vi "BER_Graphic.vi"(4 "Window Size":dbl=30.0, 5 "Instantaneous BER":dbl) -> (2 "Graph Instantaneous BER":dbl)   [LabVIEW 2022 SP3]
uses:
  <vilib>/Analysis/baseanly.llb/Mean (DBL).vi
  <vilib>/Analysis/NI_AALBase.lvlib
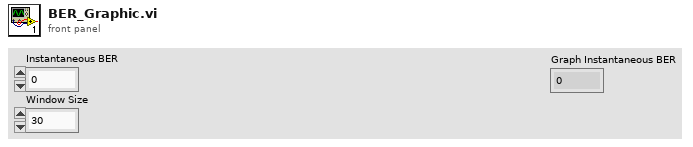
[diagram p1: front panel]
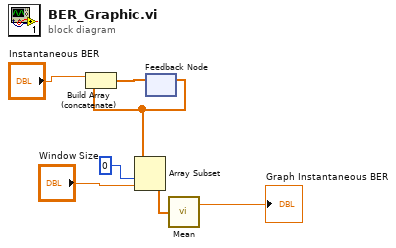
[diagram p0: block diagram]
diagram:
  n1 = feedback #1() -> (w6:dbl[])  [unwired: 1 in]
  n2 = Build Array (concatenate)("Instantaneous BER", w6) -> (w7:dbl[])
  n3 = Array Subset(array=w6, index=0, length="Window Size") -> (w5:dbl[])
  n4 = feedback-in #1(w7) -> ()
  n5 = call-poly <vilib>:"Mean.vi"("X"=w5) -> ("mean"=→"Graph Instantaneous BER":dbl)  [unwired: 1 out]
